vi "Perform Action on Target.vi"(7 "Target Identifier":string, 8 "Error In":errorcluster, 11 "reference in":refnum<class "Measure and Stimulus Subsystems.lvclass">) -> (0 "Error Out":errorcluster, 2 "Output":variant, 3 "reference out":refnum<class "Measure and Stimulus Subsystems.lvclass">)   [LabVIEW 2023, in "HAL GOOP4.lvlib" / "Measure and Stimulus Subsystems.lvclass"]
uses:
  Measure and Stimulus Subsystems.lvclass
  Measure and Stimulus Subsystems.lvclass/Measure and Stimulus Subsystems.ctl
  <vilib>/ErrorRing/Error Ring.xnode
  <vilib>/Utility/error.llb/Error Cluster From Error Code.vi
  Interfaces/IInstrument/IInstrument.lvclass
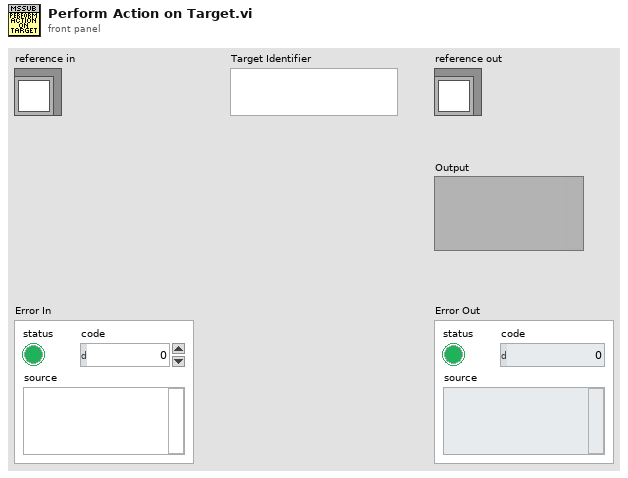
[diagram p1: front panel]
types:
  T1 = typedef "HAL GOOP4.lvlib/Measure and Stimulus Subsystems.lvclass/ObjectAttributes.ctl" = cluster{"Virt Instr":map{string, cluster{"IInstrument Base":refnum<class "IInstrument.lvclass">, "Channel":u8}}, "Physical Instr":map{string, cluster{"IInstrument Base":refnum<class "IInstrument.lvclass">, "Ref Count":u8}}}
  T2 = map{string, cluster{"IInstrument Base":refnum<class "IInstrument.lvclass">, "Ref Count":u8}}
  T3 = map{string, cluster{"Instr Identifier":string, "Channel":u8, "Perform Action Class":string}}
  T4 = cluster{"Instr Identifier":string, "Channel":u8, "Perform Action Class":string}
  T5 = cluster{"IInstrument Base":refnum<class "IInstrument.lvclass">, "Ref Count":u8}
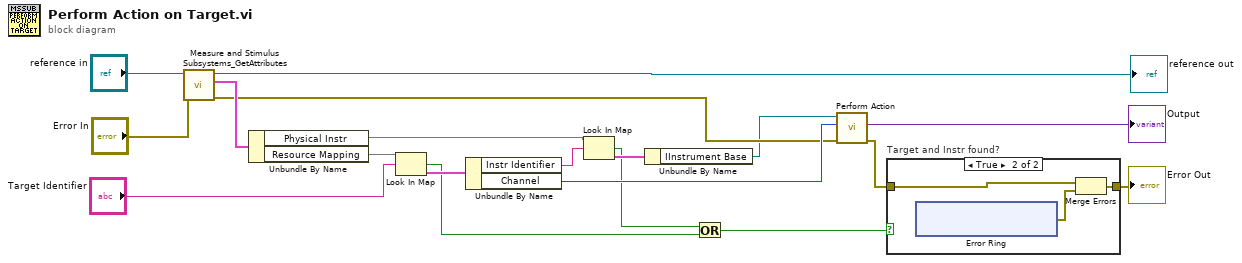
[diagram p0: block diagram]
diagram:
  n1 = call "Measure and Stimulus Subsystems_GetAttributes.vi"("Error In"="Error In", "reference in"="reference in") -> ("Error Out"=w7:errorcluster, "Data"=w11:T1, "reference out"=→"reference out":refnum<class "Measure and Stimulus Subsystems.lvclass">)  [unwired: 6 in, 1 out]
  n2 = Unbundle By Name(w11) -> ("Physical Instr"=w10:T2, "Resource Mapping"=w14:T3)
  n3 = Look In Map(map=w14, key="Target Identifier") -> (key not found?=w5:bool, value=w13:T4)  [unwired: 1 in]
  n4 = Unbundle By Name(w13) -> ("Instr Identifier"=w9:string, "Channel"=w12:u8)
  n5 = Look In Map(map=w10, key=w9) -> (key not found?=w6:bool, value=w8:T5)  [unwired: 1 in]
  n6 = Unbundle By Name(w8) -> ("IInstrument Base"=w1:refnum<class "IInstrument.lvclass">)
  n7 = Or(x=w6, y=w5) -> (x .or. y?=w4:bool)
  n8 = call-dynamic "Perform Action.vi"("Error In"=w7, "Input"=w12, "object in"=w1) -> ("Error Out"=w3:errorcluster, "Output"=→"Output":variant)  [unwired: 6 in, 1 out]
  n9 = case "Target and Instr found?" shown="True" w4 {
    tunnel: w3 -> [w20 w22]
    tunnel: [w20 w21] -> w2
    frame False {
    }
    frame True {
      n10 = xnode "Error Ring"() -> ("error out"=w23:errorcluster)
      n11 = Merge Errors(w22, w23) -> (w21:errorcluster)
    }
  }
  "Error Out" <- w2
